vi "PhysioMoment.vi"() -> ()   [LabVIEW 2012]
doc: "Demonstrates general use of Obtain Queue, queues and the effects different settings have on queue behavior. It uses a queue to pass data between an Enqueue loop (producing data) and a Dequeue loop (consuming data). If both loops run at the same speed, the queue does not fill up.\n\nWhen the Enqueue loop runs fast and the Dequeue loop runs slow, the queue quickly fills up and the Enqueue loop must wait for the Dequeue loop to remove elements. If the Enqueue loop runs slow and the Dequeue loop runs fast, the queue is quickly emptied and the Dequeue loop must wait for the Enqueue loop to insert elements."
uses:
  global_variable/tvi_arx_ni9234_global.vi
  <vilib>/Utility/file.llb/Read From Spreadsheet File (I64).vi
  <vilib>/Utility/file.llb/Read From Spreadsheet File (DBL).vi
  <vilib>/Analysis/2dsp.llb/Decimate (continuous, DBL).vi
  <vilib>/Analysis/baseanly.llb/Mean (DBL).vi
  <vilib>/Utility/file.llb/Write To Spreadsheet File (DBL).vi
  <vilib>/Analysis/NI_AALBase.lvlib
  <vilib>/Analysis/NI_AALPro.lvlib
panel:
  in  "ECG":T1={"AMP."=1.0, "high cutoff"=0.0, "low cutoff"=0.0} {"low cutoff" format="%0.4f"; "high cutoff" format="%0.2f"}
  in  "LoadCell (4)":T1={"AMP."=1.0, "high cutoff"=0.0, "low cutoff"=0.0} {"low cutoff" format="%0.4f"; "high cutoff" format="%0.2f"}
  in  "LoadCell (3)":T1={"AMP."=1.0, "high cutoff"=0.0, "low cutoff"=0.0} {"low cutoff" format="%0.4f"; "high cutoff" format="%0.2f"}
  in  "LoadCell (2)":T1={"AMP."=1.0, "high cutoff"=0.0, "low cutoff"=0.0} {"low cutoff" format="%0.4f"; "high cutoff" format="%0.2f"}
  in  "LoadCell (1)":T1={"AMP."=1.0, "high cutoff"=0.0, "low cutoff"=0.0} {"low cutoff" format="%0.4f"; "high cutoff" format="%0.2f"}
  out "file length":i32=921600
  out "output data size":i32
  out "transfer data size":i32
  out "transfer data":csg[](array[numeric])
  in  "Tab Control 2":enum32{"Settings", "Main Panel"}(tab)
  in  "Hours":i32
  in  "minutes":i32=14
  in  "seconds":i32
  in  "Led Runner File":path=path "C:/Documents and Settings/nn4080/桌面/biofeedback system/control_file/led_pixel_7phase.txt"
  in  "Led Text File":path=path "C:/Documents and Settings/nn4080/桌面/biofeedback system/control_file/Led_like.txt"
  in  "Transfer Function":path=path "C:/Documents and Settings/nn4080/桌面/biofeedback system/control_file/FFT_512hzx10sec_modeling.txt"
  in  "Name":string
  out "ECG File":path=path "D:/PVDF-ACC-0102-1013.txt"
  out "GRF File":path=path "D:/PVDF-ACC-0102-1013.txt"
  out "CURRENT STEP INTERVAL (sec)":dbl format="%#_3g"
  out "Recording":bool
  out "Boolean 2":bool
  out "Hours":i32
  out "minutes":i32=30
  out "seconds":i32
  in  "stop":bool
  in  "Tab Control":enum32{"GRF", "Raw Data"}(tab)
  out "10 SLOPE INCREMENT":dbl format="%#_3g"
  out "10 STRIDE INCREMENT":dbl format="%#_3g"
  out "5 SLOPE INCREMENT":dbl format="%#_3g"
  out "5 STRIDE INCREMENT":dbl format="%#_3g"
  out "1 SLOPE INCREMENT":dbl format="%#_3g"
  out "1 STRIDE INCREMENT":dbl format="%#_3g"
  out "TVItv SCORE":dbl format="%#_3g"
  out "Slope SCORE":dbl format="%#_3g"
  out "TVItv SCORE":dbl format="%#_3g"
  out "Slope SCORE":dbl format="%#_3g"
  out "Slope SCORE":dbl format="%#_3g"
  out "TVItv SCORE":dbl format="%#_3g"
  out "Bio-Feedback System":bool[][](array[boolean])
  out "Right Foot GRF":cluster{dbl[], "Z-Score":dbl[]}[](graph)
  out "Left Foot GRF":cluster{dbl[], "Z-Score":dbl[]}[](graph)
  out "1 Stride":cluster{i32[], "Best Linear Fit":dbl[]}[](graph)
  out "5 Strides":cluster{i32[], "Best Linear Fit":dbl[]}[](graph)
  out "10 Strides":cluster{i32[], "Best Linear Fit":dbl[]}[](graph)
  out "GRF Output":dbl[](graph)
  out "GRF Input":cluster{dbl[], "Z-Score":dbl[]}[](graph)
  out "ECG":dbl[](graph)
  out "led loop execute time":dbl
  out "tvit (10 strides)":dbl
  out "tvit (10 strides)":dbl[](array[numeric])
  out "running phase":i8
  out "step-interval":dbl
  out "baseline value":dbl
  out "tvit array size\n(step count)":i32
  out "tvit (step)":dbl[](array[numeric])
  out "tvit (stride)":dbl
  out "tvit stride":dbl[](array[numeric])
  out "tvit stride array size":i32
  out "tvit (5 strides)":dbl[](array[numeric])
  out "tvit (5 strides)":dbl
  out "mean":dbl
  out "new step interval":dbl
  out "new step global index":dbl
  out "Tvit of new step":dbl
  out "step-index":dbl[](array[numeric])
  out "step-length":dbl[](array[numeric])
  out "vaild Tvit":dbl[](array[numeric])
  out "points per loop":i32
  out "GRF Input size":i32
  out "GRF Output size":i32
  out "main loop":i32
  out "std(loadcell)":dbl
  out "new step index(global) in last loop":dbl
  out "window start index":i32
  out "new step interval in last loop":dbl
  out "counter (sec)":string
  out "loop execution time":dbl
  out "zero-crossing point\n(increasing)":dbl[](array[numeric])
  out "area between zero-crossing points \n(z-score series)":dbl[](array[numeric])
  out "interval between \nzero-crossing points":dbl[](array[numeric])
  out "zero-crossing interval\nlower threshold":dbl
  out "step-index\n(in window)":dbl[](array[numeric])
  # "Ground Reaction Force \nBio-FeedBack System"
  # "Setting Time"
  # "Elapsed Time"
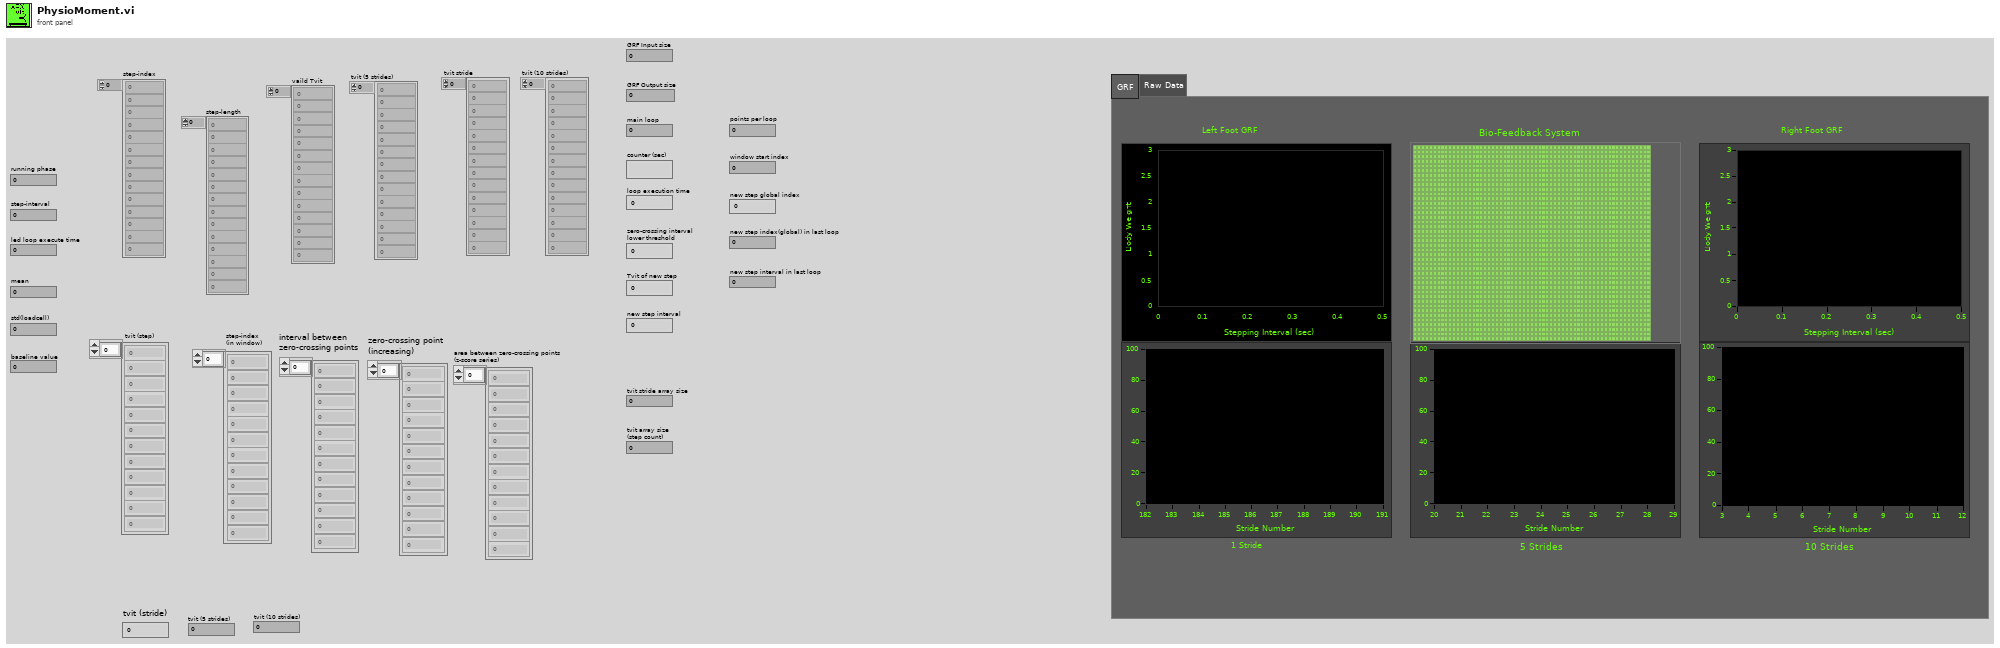
[diagram p1: front panel]
types:
  T1 = cluster{"AMP.":dbl, "high cutoff":dbl, "low cutoff":dbl}
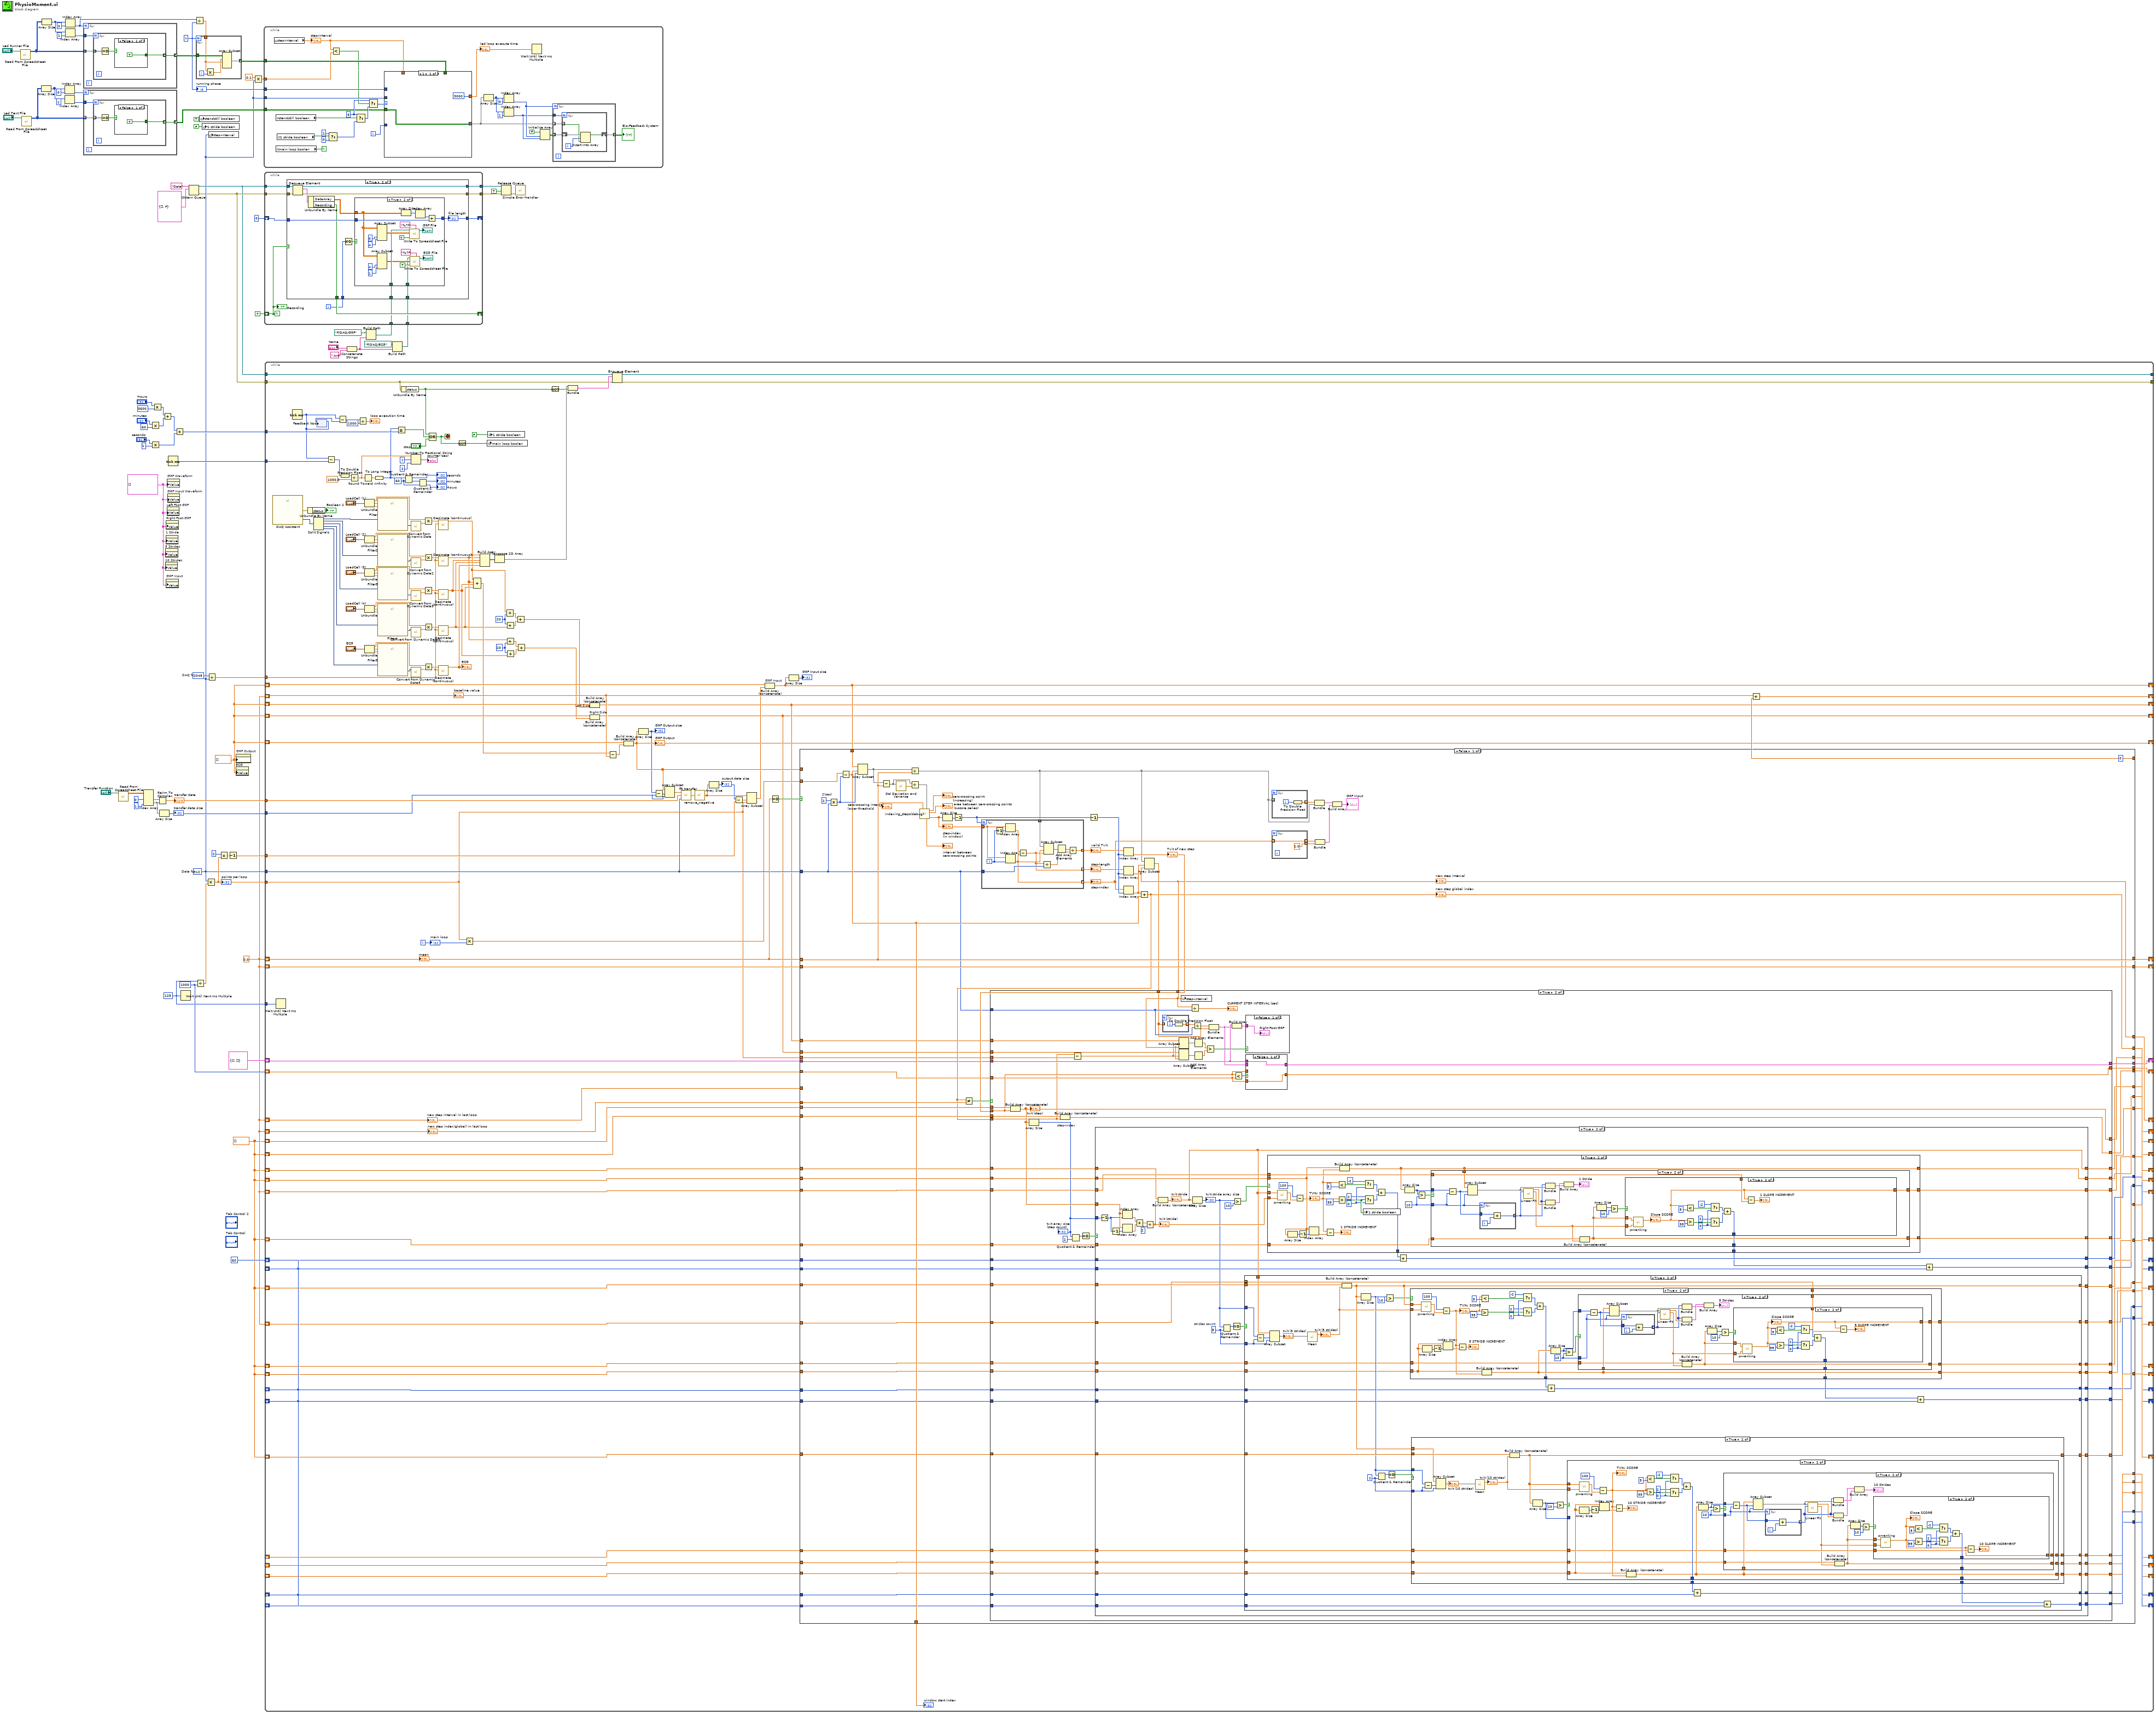
[diagram p0: block diagram]
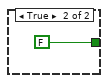
[diagram p4: hidden frame]
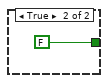
[diagram p5: hidden frame]
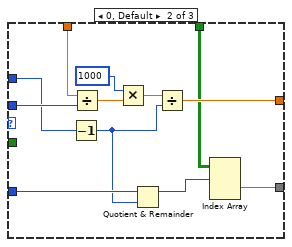
[diagram p6: hidden frame]
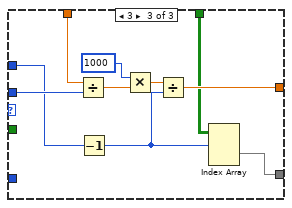
[diagram p7: hidden frame]
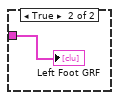
[diagram p10: hidden frame]
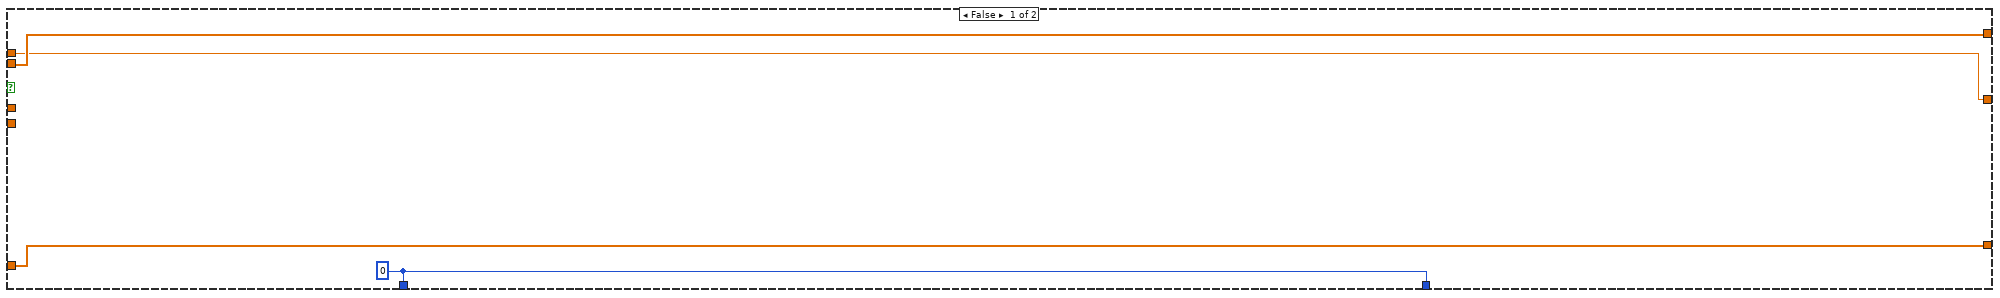
[diagram p12: hidden frame]
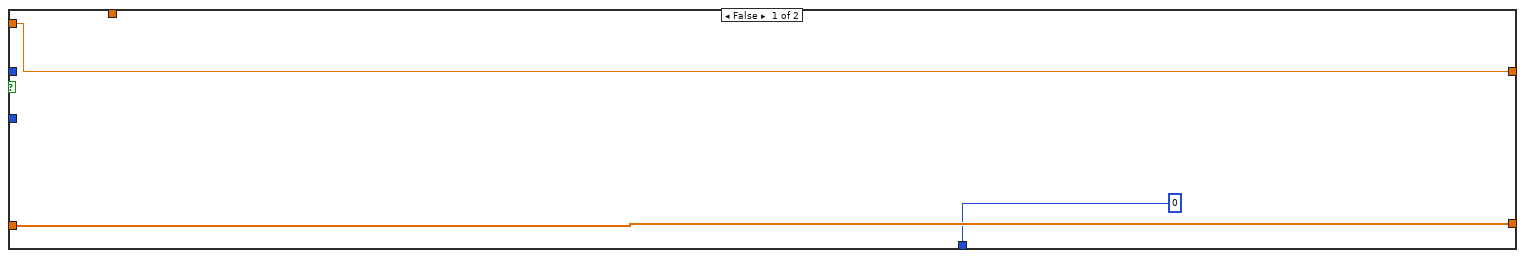
[diagram p13: hidden frame]
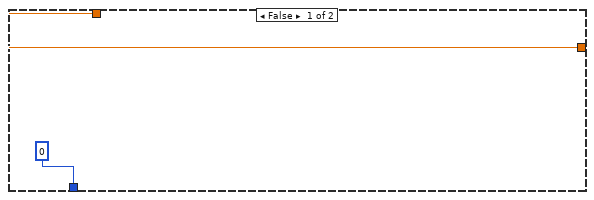
[diagram p14: hidden frame]
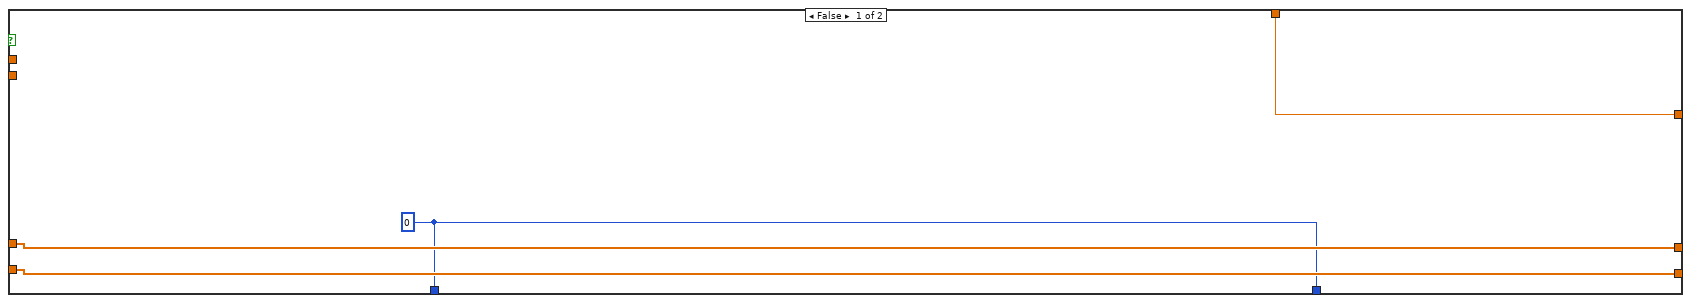
[diagram p16: hidden frame]
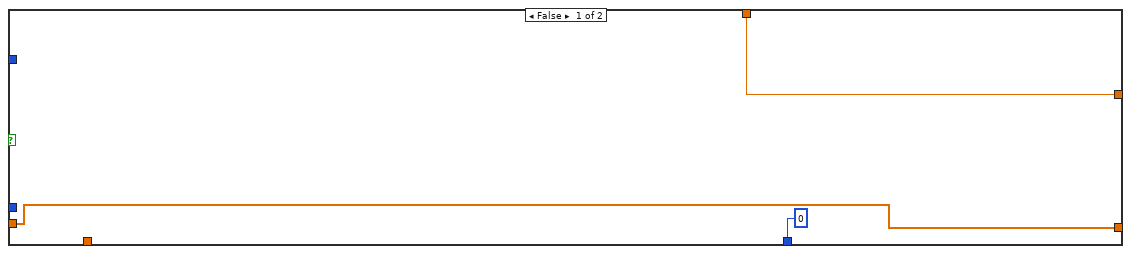
[diagram p17: hidden frame]
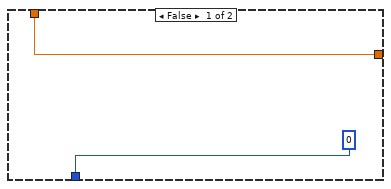
[diagram p18: hidden frame]
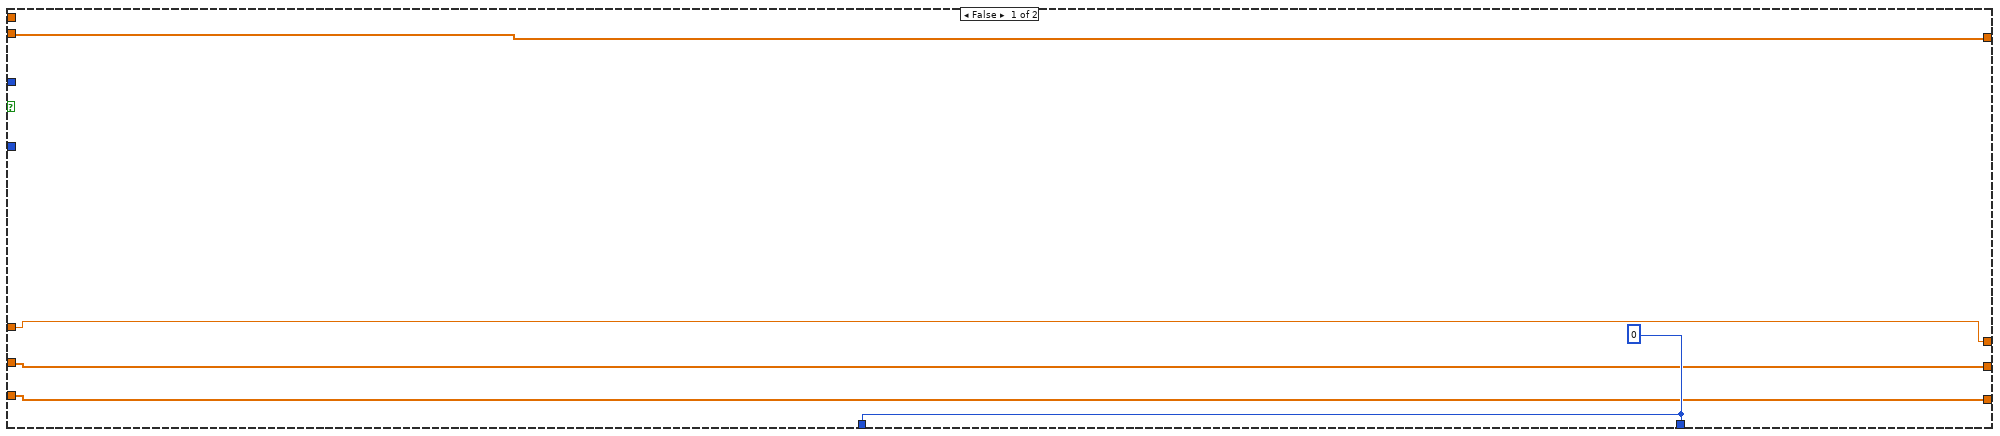
[diagram p19: hidden frame]
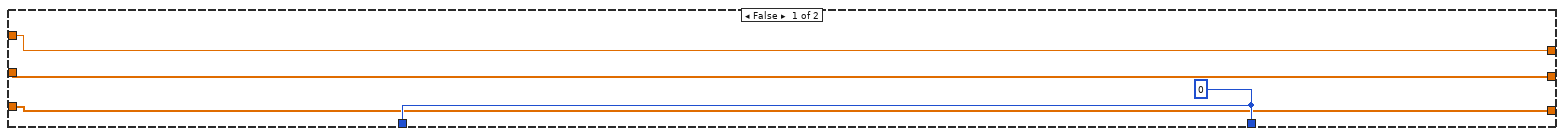
[diagram p20: hidden frame]
diagram:
  w9 = 2048  # DAQ fs
  w39 = 60
  (unwired) 1
  w41 = 7
  w1 = dbl[] []
  w4 = cluster{dbl[], "Z-Score":dbl[]}[] [] ("Z-Score Waveform (2 sec)")
  w2 = 0.0
  w8 = 512  # Data fs
  w3 = dbl[] []
  w31 = 1000
  w63 = u32 125 ("millisecond multiple")
  n1 = call-poly <vilib>:"Read From Spreadsheet File.vi"("file path (dialog if empty)"="Led Runner File") -> ("all rows"=w52:i64[][])  [unwired: 6 in, 4 out]
  n2 = call-poly <vilib>:"Read From Spreadsheet File.vi"("file path (dialog if empty)"="Led Text File") -> ("all rows"=w46:i64[][])  [unwired: 6 in, 4 out]
  n3 = Array Size(array=w46) -> (size(s)=w47:i32[])
  n4 = Array Size(array=w52) -> (size(s)=w51:i32[])
  n5 = Index Array(array=w47, index=0) -> (element=w45:i32)
  n6 = Index Array(array=w47) -> (element=w44:i32)  [unwired: 1 in]
  n7 = Index Array(array=w51, index=0) -> (element=w42:i32)
  n8 = Index Array(array=w51, index=1) -> (element=w55:i32)
  n9 = for {
    N: w42 -> [_]
    tunnel: w52 -> [w78] mode=indexing
    tunnel: [w77] -> w54 mode=indexing
    tunnel: w55 -> [w76]
    n10 = for {
      N: w76 -> [_]
      tunnel: w78 -> [w80] mode=indexing
      tunnel: [w79] -> w77 mode=indexing
      n11 = Equal To 0?(x=w80) -> (x = 0?=w81:bool)
      n12 = case shown="False" w81 {
        tunnel: [TRUE FALSE] -> w79
        frame False {
        }
        frame True {
        }
      }
    }
  }
  n13 = for {
    N: w45 -> [_]
    tunnel: w46 -> [w86] mode=indexing
    tunnel: [w85] -> w43 mode=indexing
    tunnel: w44 -> [w84]
    n14 = for {
      N: w84 -> [_]
      tunnel: w86 -> [w88] mode=indexing
      tunnel: [w87] -> w85 mode=indexing
      n15 = Equal To 0?(x=w88) -> (x = 0?=w89:bool)
      n16 = case shown="False" w89 {
        tunnel: [TRUE FALSE] -> w87
        frame False {
        }
        frame True {
        }
      }
    }
  }
  n17 = call-poly <vilib>:"Read From Spreadsheet File.vi"("file path (dialog if empty)"="Transfer Function") -> ("all rows"=w37:dbl[][])  [unwired: 6 in, 4 out]
  n18 = Index Array(array=w37, index (col) #1=0, index (col) #2=1) -> (element #1=w34:dbl[], element #2=w32:dbl[])  [unwired: 2 in]
  n19 = Multiply(x="minutes", y=60) -> (x*y=w75:i32)
  n20 = Multiply(x="seconds", y=1) -> (x*y=w66:i32)
  n21 = Multiply(x="Hours", y=3600) -> (x*y=w74:i32)
  n22 = Re/Im To Complex(1:w32, 2:w34) -> (0:w33:cdb[])
  "transfer data" <- w33
  n23 = Array Size(array=w32) -> (size(s)=w27:i32)
  "transfer data size" <- w27
  n24 = Add(x=w74, y=w75) -> (x+y=w67:i32)
  n25 = property on="10 Strides" class="XYGraph (strict)"("Value"=w4) -> ()  [unwired: 2 in, 2 out]
  n26 = property on="5 Strides" class="XYGraph (strict)"("Value"=w4) -> ()  [unwired: 2 in, 2 out]
  n27 = property on="1 Stride" class="XYGraph (strict)"("Value"=w4) -> ()  [unwired: 2 in, 2 out]
  n28 = property on="Right Foot GRF" class="XYGraph (strict)"("Value"=w4) -> ()  [unwired: 2 in, 2 out]
  n29 = property on="GRF Input" class="XYGraph (strict)"("Value"=w4) -> ()  [unwired: 2 in, 2 out]
  n30 = property on="Left Foot GRF" class="XYGraph (strict)"("Value"=w4) -> ()  [unwired: 2 in, 2 out]
  n31 = property on="GRF Waveform" class="XYGraph (strict)"("Value"=w4) -> ()  [unwired: 2 in, 2 out]
  n32 = property on="GRF Input Waveform" class="XYGraph (strict)"("Value"=w4) -> ()  [unwired: 2 in, 2 out]
  n33 = Tick Count (ms)() -> (millisecond timer value=w65:u32)
  n34 = Add(x=w67, y=w66) -> (x+y=w64:i32)
  n35 = Wait Until Next ms Multiple(millisecond multiple=w63) -> ()  [unwired: 1 out]
  n36 = Obtain Queue(name (unnamed)="Data", element data type=cluster{"DataArray":dbl[][], "Recording":bool} {"DataArray"=[], "Recording"=FALSE}) -> (queue out=w5:refnum<queue>, error out=w6:errorcluster)  [unwired: 3 in, 1 out]
  n37 = Divide(x=w42, y=w41) -> (x/y=w40:dbl)
  n38 = Divide(x=w63, y=w31) -> (x/y=w62:dbl)
  n39 = for {
    N: w41 -> [_]
    tunnel: w54 -> [w96]
    tunnel: w40 -> [w93]
    tunnel: [w94] -> w53 mode=indexing
    i -> [w95]
    n40 = Multiply(x=w93, y=w95) -> (x*y=w92:dbl)
    n41 = Array Subset(array=w96, index (row)=w92, length (row)=w93) -> (w94:bool[][])  [unwired: 2 in]
  }
  n42 = global write "tvi_arx_ni9234_global.vi" "standstill boolean"(TRUE) -> ()
  n43 = global write "tvi_arx_ni9234_global.vi" "1 stride boolean"(FALSE) -> ()
  n44 = Multiply(x=w8, y=w62) -> (x*y=w28:dbl)
  "points per loop" <- w28
  n45 = Divide(x=w9, y=w8) -> (x/y=w7:dbl)
  n46 = global write "tvi_arx_ni9234_global.vi" "step-interval"(w8) -> ()
  n47 = Multiply(x=2, y=w28) -> (x*y=w26:dbl)
  n48 = Decrement(x=w26) -> (x-1=w25:dbl)
  n49 = property on="GRF Output" class="WFChart (strict)"("History Data"=w3) -> ()  [unwired: 2 in, 2 out]
  n50 = property on="ECG" class="WFChart (strict)"("Value"=w3) -> ()  [unwired: 2 in, 2 out]
  n51 = Multiply(x=0.1, y=w8) -> (x*y=w49:dbl)
  n52 = while {
    tunnel: w53 -> [w118]
    tunnel: w8 -> [w116]
    tunnel: w41 -> [w119]
    tunnel: w49 -> [w103]
    tunnel: w43 -> [w98]
    i -> [w120]
    stop <- w123 continue-if-true
    w100 = 3
    n53 = global read "tvi_arx_ni9234_global.vi" "step-interval"() -> (w104:dbl)
    "step-interval" <- w104
    n54 = global read "tvi_arx_ni9234_global.vi" "standstill boolean"() -> (w114:bool)
    n55 = global read "tvi_arx_ni9234_global.vi" "main loop boolen"() -> (w123:bool)
    n56 = global read "tvi_arx_ni9234_global.vi" "1 stride boolean"() -> (w117:bool)
    n57 = Select(t=1, s=w117, f=0) -> (s? t:f=w97:i32)
    n58 = Less?(x=w104, y=w103) -> (x < y?=w102:bool)
    n59 = Select(t=w100, s=w114, f=w97) -> (s? t:f=w99:i32)
    n60 = Select(t=w100, s=w102, f=w99) -> (s? t:f=w101:i32)
    n61 = case shown="1" w101 {
      tunnel: w120 -> [_ w145 _]
      tunnel: w119 -> [_ w138 w149]
      tunnel: w118 -> [_ w136 w147]
      tunnel: w116 -> [_ w141 w151]
      tunnel: w104 -> [_ w140 w152]
      tunnel: [3000 w139 w150] -> w115
      tunnel: [w132 w134 w148] -> w105
      tunnel: w98 -> [w132 _ _]
      frame 1 {
      }
      frame 0, Default {
        n62 = Decrement(x=w138) -> (x-1=w137:i32)
        n63 = Divide(x=w140, y=w141) -> (x/y=w143:dbl)
        n64 = Multiply(x=1000, y=w143) -> (x*y=w144:dbl)
        n65 = Quotient & Remainder(x=w145, y=w137) -> (x-y*floor(x/y)=w135:i32)  [unwired: 1 out]
        n66 = Divide(x=w144, y=w137) -> (x/y=w139:dbl)
        n67 = Index Array(array=w136, index (dim 0)=w135) -> (element=w134:bool[][])  [unwired: 2 in]
      }
      frame 3 {
        n68 = Divide(x=w152, y=w151) -> (x/y=w154:dbl)
        n69 = Decrement(x=w149) -> (x-1=w146:i32)
        n70 = Multiply(x=1000, y=w154) -> (x*y=w155:dbl)
        n71 = Divide(x=w155, y=w146) -> (x/y=w150:dbl)
        n72 = Index Array(array=w147, index (dim 0)=w146) -> (element=w148:bool[][])  [unwired: 2 in]
      }
    }
    "led loop execute time" <- w115
    n73 = Array Size(array=w105) -> (size(s)=w108:i32[])
    n74 = Index Array(array=w108, index=0) -> (element=w107:i32)
    n75 = Index Array(array=w108, index=1) -> (element=w106:i32)
    n76 = Wait Until Next ms Multiple(millisecond multiple=w115) -> ()  [unwired: 1 out]
    n77 = Initialize Array(FALSE, w107, w106) -> (w112:bool[][])
    n78 = for {
      N: w107 -> [_]
      tunnel: [w127] -> w109 mode=indexing
      tunnel: w105 -> [w126] mode=indexing
      tunnel: w112 -> [w125] mode=indexing
      tunnel: w106 -> [w124]
      n79 = for {
        N: w124 -> [_]
        tunnel: w126 -> [w128] mode=indexing
        shift-right: [w131] -> w127
        shift-left: w125 -> [w129]
        i -> [w130]
        n80 = Insert Into Array(array=w129, index=w130, new element=w128) -> (w131:bool[])
      }
    }
    "Bio-Feedback System" <- w109
  }
  n81 = while {
    tunnel: w65 -> [w324]
    tunnel: w64 -> [w323]
    tunnel: w63 -> [w320]
    shift-right: [w282] -> _
    shift-left: w2 -> [w292]
    shift-right: [w281] -> _
    shift-left: w2 -> [w291]
    tunnel: w28 -> [w156]
    shift-right: [w243] -> _
    shift-left: w3 -> [w307]
    tunnel: w8 -> [w242]
    shift-right: [w286] -> _
    shift-left: w3 -> [w306]
    shift-right: [w302] -> _
    shift-left: w2 -> [w303]
    shift-right: [w301] -> _
    shift-left: w2 -> [w300]
    shift-right: [w285] -> _
    shift-left: w1 -> [w298]
    shift-right: [w284] -> _
    shift-left: w1 -> [w297]
    shift-right: [w296] -> _
    shift-left: w1 -> [w295]
    shift-right: [w294] -> _
    shift-left: w1 -> [w293]
    shift-right: [w288] -> _
    shift-left: w2 -> [w287]
    shift-right: [w279] -> _
    shift-left: w1 -> [w278]
    shift-right: [w276] -> _
    shift-left: w1 -> [w275]
    shift-right: [w274] -> _
    shift-left: w39 -> [w273]
    shift-right: [w272] -> _
    shift-left: w39 -> [w269]
    shift-right: [w271] -> _
    shift-left: w1 -> [w270]
    shift-right: [w268] -> _
    shift-left: w1 -> [w267]
    shift-right: [w266] -> _
    shift-left: w39 -> [w265]
    shift-right: [w262] -> _
    shift-left: w39 -> [w261]
    shift-right: [w264] -> _
    shift-left: w1 -> [w263]
    shift-right: [w260] -> _
    shift-left: w39 -> [w254]
    shift-right: [w259] -> _
    shift-left: _ -> [w258]
    shift-right: [w257] -> _
    shift-left: _ -> [w256]
    shift-right: [w255] -> _
    shift-left: w39 -> [w253]
    shift-right: [w252] -> _
    shift-left: _ -> [w251]
    shift-right: [w250] -> _
    shift-left: w2 -> [w249]
    shift-right: [w248] -> _
    shift-left: w2 -> [w247]
    tunnel: w33 -> [w244]
    tunnel: w27 -> [w238]
    shift-right: [w223] -> _
    shift-left: w3 -> [w227]
    shift-right: [w222] -> _
    shift-left: w3 -> [w226]
    shift-right: [w218] -> _
    shift-left: cluster{dbl[], dbl[]} {[], []} -> [w221]
    shift-right: [w219] -> _
    shift-left: w31 -> [w220]
    tunnel: w25 -> [w217]
    tunnel: w7 -> [w170]
    tunnel: [w163] -> _
    tunnel: [w162] -> _
    tunnel: w5 -> [w159]
    tunnel: w6 -> [w158]
    i -> [w157]
    stop <- w283 stop-if-true
    w228 = 20
    w229 = 20
    w299 = 60 ("floor(x/y)")
    n82 = call "DAQ Assistant"() -> ("data"=w201:dynamicdata, "error out"=w216:errorcluster)  [unwired: 16 in, 2 out]
    n83 = Wait Until Next ms Multiple(millisecond multiple=w320) -> ()  [unwired: 1 out]
    n84 = Tick Count (ms)() -> (millisecond timer value=w311:u32)
    n85 = Unbundle By Name(w216) -> ("status"=→"Boolean 2":bool)
    n86 = Split Signals(w201) -> (w200:dynamicdata, w199:dynamicdata, w176:dynamicdata, w175:dynamicdata, w174:dynamicdata)  [unwired: 5 in]
    n87 = feedback-in #1(w311) -> ()
    n88 = feedback #1() -> (w316:u32)  [unwired: 1 in]
    n89 = Subtract(x=w311, y=w324) -> (x-y=w326:u32)
    n90 = Subtract(x=w311, y=w316) -> (x-y=w319:u32)
    n91 = To Double Precision Float(number=w326) -> (double precision float=w327:dbl)
    n92 = Divide(x=w327, y=1000.0) -> (x/y=w312:dbl)
    n93 = Divide(x=w319, y=1000) -> (x/y=→"loop execution time":dbl)
    n94 = Round Toward -Infinity(1:w312) -> (0:w325:dbl)
    n95 = Unbundle("LoadCell (1)") -> ("AMP."=w207:dbl, "high cutoff"=w213:dbl, "low cutoff"=w212:dbl)
    n96 = Unbundle("LoadCell (2)") -> ("AMP."=w204:dbl, "high cutoff"=w211:dbl, "low cutoff"=w210:dbl)
    n97 = Unbundle("LoadCell (3)") -> ("AMP."=w188:dbl, "high cutoff"=w194:dbl, "low cutoff"=w193:dbl)
    n98 = Unbundle("LoadCell (4)") -> ("AMP."=w185:dbl, "high cutoff"=w192:dbl, "low cutoff"=w191:dbl)
    n99 = Unbundle("ECG") -> ("AMP."=w173:dbl, "high cutoff"=w181:dbl, "low cutoff"=w180:dbl)
    n100 = To Long Integer(number=w325) -> (32bit integer=w309:i32)
    n101 = call "Filter"("Lower Cut-Off"=w212, "Upper Cut-Off"=w213, "Signal"=w200) -> ("Filtered Signal"=w209:dynamicdata)  [unwired: 7 in, 1 out]
    n102 = call "Filter2"("Lower Cut-Off"=w210, "Upper Cut-Off"=w211, "Signal"=w199) -> ("Filtered Signal"=w205:dynamicdata)  [unwired: 7 in, 1 out]
    n103 = call "Filter3"("Lower Cut-Off"=w193, "Upper Cut-Off"=w194, "Signal"=w176) -> ("Filtered Signal"=w190:dynamicdata)  [unwired: 7 in, 1 out]
    n104 = call "Filter4"("Lower Cut-Off"=w191, "Upper Cut-Off"=w192, "Signal"=w175) -> ("Filtered Signal"=w186:dynamicdata)  [unwired: 7 in, 1 out]
    n105 = call "Filter5"("Lower Cut-Off"=w180, "Upper Cut-Off"=w181, "Signal"=w174) -> ("Filtered Signal"=w178:dynamicdata)  [unwired: 7 in, 1 out]
    n106 = Greater Or Equal?(x=w309, y=w323) -> (x >= y?=w322:bool)
    n107 = Unbundle By Name(w158) -> ("status"=w160:bool)
    n108 = Quotient & Remainder(x=w309, y=w299) -> (x-y*floor(x/y)=→"seconds":i32, floor(x/y)=w328:i32)
    n109 = call "Convert from Dynamic Data"("Dynamic Data Type"=w209) -> ("Array"=w208:dbl[])  [unwired: 3 in]
    n110 = call "Convert from Dynamic Data2"("Dynamic Data Type"=w205) -> ("Array"=w206:dbl[])  [unwired: 3 in]
    n111 = call "Convert from Dynamic Data3"("Dynamic Data Type"=w190) -> ("Array"=w189:dbl[])  [unwired: 3 in]
    n112 = call "Convert from Dynamic Data4"("Dynamic Data Type"=w186) -> ("Array"=w187:dbl[])  [unwired: 3 in]
    n113 = call "Convert from Dynamic Data5"("Dynamic Data Type"=w178) -> ("Array"=w179:dbl[])  [unwired: 3 in]
    n114 = Number To Fractional String(number=w312, width (-)=7, precision (6)=2) -> (F-format string=→"counter (sec)":string)  [unwired: 1 in]
    n115 = Quotient & Remainder(x=w328, y=w299) -> (x-y*floor(x/y)=→"minutes":i32, floor(x/y)=→"Hours":i32)
    n116 = Multiply(x=w207, y=w208) -> (x*y=w198:dbl[])
    n117 = Multiply(x=w188, y=w189) -> (x*y=w184:dbl[])
    n118 = Multiply(x=w204, y=w206) -> (x*y=w197:dbl[])
    n119 = Multiply(x=w185, y=w187) -> (x*y=w183:dbl[])
    n120 = Multiply(x=w173, y=w179) -> (x*y=w177:dbl[])
    n121 = Compound Arithmetic op=OR(w160, w322, "stop") -> (w283:bool)
    n122 = call-poly <vilib>:"Decimate (continuous).vi"("decimating factor"=w170, "X"=w198) -> ("Decimated Array"=w168:dbl[])  [unwired: 8 in, 1 out]
    n123 = call-poly <vilib>:"Decimate (continuous).vi"("decimating factor"=w170, "X"=w197) -> ("Decimated Array"=w167:dbl[])  [unwired: 8 in, 1 out]
    n124 = call-poly <vilib>:"Decimate (continuous).vi"("decimating factor"=w170, "X"=w184) -> ("Decimated Array"=w166:dbl[])  [unwired: 8 in, 1 out]
    n125 = call-poly <vilib>:"Decimate (continuous).vi"("decimating factor"=w170, "X"=w183) -> ("Decimated Array"=w169:dbl[])  [unwired: 8 in, 1 out]
    n126 = call-poly <vilib>:"Decimate (continuous).vi"("decimating factor"=w170, "X"=w177) -> ("Decimated Array"=w172:dbl[])  [unwired: 8 in, 1 out]
    "ECG" <- w172
    n127 = Not(x=w283) -> (.not. x?=w280:bool)
    n128 = Multiply(x=w156, y=w157) -> (x*y=w241:dbl)
    n129 = Compound Arithmetic op=ADD(w168, w167, w166, w169) -> (w171:dbl[])
    n130 = Build Array(w168, w167, w166, w169, w172) -> (w202:dbl[][])
    n131 = global write "tvi_arx_ni9234_global.vi" "main loop boolen"(w280) -> ()
    n132 = global write "tvi_arx_ni9234_global.vi" "1 stride boolean"(FALSE) -> ()
    n133 = Transpose 2D Array(2D array=w202) -> (transposed array=w161:dbl[][])
    n134 = Add(x=w168, y=w228) -> (x+y=w231:dbl[])
    n135 = Add(x=w228, y=w169) -> (x+y=w230:dbl[])
    n136 = Add(x=w167, y=w229) -> (x+y=w233:dbl[])
    n137 = Add(x=w229, y=w166) -> (x+y=w232:dbl[])
    n138 = Add(x=w231, y=w230) -> (x+y=w225:dbl[])
    n139 = Add(x=w233, y=w232) -> (x+y=w224:dbl[])
    n140 = Not(x=w160) -> (.not. x?=w165:bool)
    n141 = Bundle(w161, w165) -> (w164:cluster{dbl[][], bool})  [unwired: 1 in]
    n142 = Build Array (concatenate) "Right Side"(w226, w224) -> (w222:dbl[])
    n143 = Build Array (concatenate) "Left Side"(w227, w225) -> (w223:dbl[])
    n144 = Subtract(x=w171, y=w287) -> (x-y=w290:dbl[])
    n145 = Enqueue Element(queue=w159, element=w164, error in (no error)=w158) -> (queue out=w163:refnum<queue>, error out=w162:errorcluster)  [unwired: 1 in, 1 out]
    n146 = Build Array (concatenate)(w307, w290) -> (w243:dbl[])
    "GRF Output" <- w243
    n147 = Array Size(array=w243) -> (size(s)=w239:i32)
    "GRF Output size" <- w239
    n148 = Subtract(x=w239, y=w238) -> (x-y=w240:i32)
    n149 = Array Subset(array=w243, index=w240, length=w238) -> (w246:dbl[])
    n150 = call "fft_transfer.vi"("Sample Rate"=w242, "Transfer Function"=w244, "GRF Output"=w246) -> ("GRF Input"=w245:dbl[])
    n151 = call "remove_negative.vi"("input array"=w245) -> ("output array"=w237:dbl[])
    n152 = Array Size(array=w237) -> (size(s)=w236:i32)
    "output data size" <- w236
    n153 = Subtract(x=w236, y=w217) -> (x-y=w235:dbl)
    n154 = Array Subset(array=w237, index=w235, length=w156) -> (w234:dbl[])
    n155 = Build Array (concatenate) "GRF Input"(w306, w234) -> (w286:dbl[])
    n156 = Equal To 0?(x=w300) -> (x = 0?=w308:bool)
    n157 = Array Size(array=w286) -> (size(s)=→"GRF Input size":i32)
    n158 = case shown="False" w308 {
      tunnel: w300 -> [w380 w943]
      tunnel: [w402 w926] -> w305
      tunnel: w242 -> [w370 w904]
      tunnel: w241 -> [w415 w924]
      tunnel: w243 -> [_ w932]
      tunnel: w303 -> [w391 w947]
      tunnel: [w391 w930] -> w302
      tunnel: [w371 w934] -> w282
      tunnel: [w375 w935] -> w281
      tunnel: [w380 w942] -> w301
      tunnel: w292 -> [w399 w934]
      tunnel: [w333 w939] -> w285
      tunnel: w298 -> [w398 w939]
      tunnel: [w397 w938] -> w284
      tunnel: w297 -> [w396 w938]
      tunnel: [w395 w937] -> w296
      tunnel: w295 -> [w394 w937]
      tunnel: [w393 w936] -> w294
      tunnel: w293 -> [w392 w936]
      tunnel: w291 -> [_ w935]
      tunnel: w286 -> [w389 w927]
      tunnel: [0 w925] -> w289
      tunnel: [w374 w923] -> w279
      tunnel: w278 -> [w373 w923]
      tunnel: [w369 w922] -> w276
      tunnel: w275 -> [w368 w922]
      tunnel: [w367 w920] -> w274
      tunnel: w273 -> [w366 w920]
      tunnel: [w365 w919] -> w272
      tunnel: [w364 w921] -> w271
      tunnel: w270 -> [w363 w921]
      tunnel: w269 -> [w362 w919]
      tunnel: [w361 w913] -> w268
      tunnel: w267 -> [w360 w913]
      tunnel: [w359 w912] -> w266
      tunnel: w265 -> [w358 w912]
      tunnel: [w357 w914] -> w264
      tunnel: w263 -> [w356 w914]
      tunnel: [w355 w911] -> w262
      tunnel: w261 -> [w354 w911]
      tunnel: [w353 w916] -> w260
      tunnel: [w352 w917] -> w259
      tunnel: w258 -> [w351 w917]
      tunnel: [w350 w918] -> w257
      tunnel: w256 -> [w349 w918]
      tunnel: [w348 w915] -> w255
      tunnel: w254 -> [w347 w916]
      tunnel: w253 -> [w346 w915]
      tunnel: [w345 w908] -> w252
      tunnel: w251 -> [w344 w908]
      tunnel: [w343 w909] -> w250
      tunnel: w249 -> [w342 w909]
      tunnel: [w341 w910] -> w248
      tunnel: w247 -> [w340 w910]
      tunnel: w223 -> [w339 _]
      tunnel: w222 -> [w338 _]
      tunnel: w221 -> [w337 w907]
      tunnel: w220 -> [w336 w906]
      tunnel: [w335 w906] -> w219
      tunnel: [w334 w907] -> w218
      tunnel: w156 -> [w332 _]
      frame False {
        w409 = 2  # 2(sec)
        n159 = Multiply(x=w409, y=w370) -> (x*y=w414:i32)
        n160 = Subtract(x=w415, y=w414) -> (x-y=w402:dbl)
        n161 = Array Subset(array=w389, index=w402, length=w414) -> (w377:dbl[])
        n162 = Subtract(x=w377, y=w380) -> (x-y=w378:dbl[])
        n163 = call <vilib>:"Std Deviation and Variance.vi"("X"=w378) -> ("standard deviation"=w416:dbl)  [unwired: 1 in, 2 out]
        n164 = Divide(x=w377, y=w380) -> (x/y=w376:dbl[])
        n165 = Divide(x=w378, y=w416) -> (x/y=w379:dbl[])
        n166 = call "indexing_steps(debug).vi"("z-score series (input)"=w379) -> ("lower threshold of zeros-interval"=→"zero-crossing interval\nlower threshold":dbl, "zeros-interval\n(interval between zero-crossing index)"=→"interval between \nzero-crossing points":dbl[], "increasing\nzero-crossing index"=→"zero-crossing point\n(increasing)":dbl[], "area between zero-crossing index"=→"area between zero-crossing points \n(z-score series)":dbl[], "index of steps (output)"=w407:dbl[])  [unwired: 1 in]
        "step-index\n(in window)" <- w407
        n167 = Array Size(array=w407) -> (size(s)=w408:i32)
        n168 = Decrement(x=w408) -> (x-1=w405:i32)
        n169 = for {
          N: w405 -> [_]
          tunnel: w407 -> [w896]
          tunnel: w376 -> [w899]
          tunnel: [w893] -> w404 mode=indexing
          tunnel: [w891] -> w403 mode=indexing
          tunnel: [w894] -> w382 mode=indexing
          tunnel: w370 -> [w895]
          i -> [w901]
          n170 = Increment(x=w901) -> (x+1=w902:i32)
          n171 = Index Array(array=w896, index=w902) -> (element=w900:dbl)
          n172 = Index Array(array=w896, index=w901) -> (element=w894:dbl)
          n173 = Subtract(x=w900, y=w894) -> (x-y=w891:dbl)
          n174 = Divide(x=w891, y=w895) -> (x/y=w892:dbl)
          n175 = Array Subset(array=w899, index=w894, length=w891) -> (w897:dbl[])
          n176 = Add Array Elements(numeric array=w897) -> (sum=w898:dbl)
          n177 = Divide(x=w898, y=w892) -> (x/y=w893:dbl)
        }
        "vaild Tvit" <- w404
        "step-length" <- w403
        "step-index" <- w382
        n178 = Decrement(x=w405) -> (x-1=w406:i32)
        n179 = Index Array(array=w404, index=w406) -> (element=w390:dbl)
        "Tvit of new step" <- w390
        n180 = Index Array(array=w403, index=w406) -> (element=w375:dbl)
        "new step interval" <- w375
        n181 = Index Array(array=w382, index=w406) -> (element=w401:dbl)
        n182 = Add(x=w401, y=w402) -> (x+y=w371:dbl)
        "new step global index" <- w371
        n183 = Not Equal?(x=w371, y=w399) -> (x != y?=w400:bool)
        n184 = Array Subset(array=w376, index=w401, length=w375) -> (w372:dbl[])
        n185 = case shown="True" w400 {
          tunnel: [w442 w498] -> w333
          tunnel: w398 -> [w442 w507]
          tunnel: w390 -> [_ w455]
          tunnel: [w440 w506] -> w397
          tunnel: w396 -> [w440 w505]
          tunnel: [w441 w504] -> w395
          tunnel: w394 -> [w441 w503]
          tunnel: [w439 w502] -> w393
          tunnel: w392 -> [w439 w501]
          tunnel: w375 -> [_ w452]
          tunnel: [w438 w500] -> w374
          tunnel: w373 -> [w438 w499]
          tunnel: w372 -> [_ w450]
          tunnel: w371 -> [_ w445]
          tunnel: w370 -> [_ w458]
          tunnel: [w437 w496] -> w369
          tunnel: w368 -> [w437 w495]
          tunnel: [w435 w494] -> w367
          tunnel: w366 -> [w435 w493]
          tunnel: [w434 w492] -> w365
          tunnel: [w436 w491] -> w364
          tunnel: w363 -> [w436 w490]
          tunnel: w362 -> [w434 w489]
          tunnel: [w432 w488] -> w361
          tunnel: w360 -> [w432 w487]
          tunnel: [w431 w486] -> w359
          tunnel: w358 -> [w431 w485]
          tunnel: [w433 w484] -> w357
          tunnel: w356 -> [w433 w483]
          tunnel: [w430 w482] -> w355
          tunnel: w354 -> [w430 w481]
          tunnel: [w427 w480] -> w353
          tunnel: [w428 w479] -> w352
          tunnel: w351 -> [w428 w478]
          tunnel: [w429 w477] -> w350
          tunnel: w349 -> [w429 w476]
          tunnel: [w426 w475] -> w348
          tunnel: w347 -> [w427 w474]
          tunnel: w346 -> [w426 w473]
          tunnel: [w423 w472] -> w345
          tunnel: w344 -> [w423 w471]
          tunnel: [w424 w470] -> w343
          tunnel: w342 -> [w424 w469]
          tunnel: [w425 w468] -> w341
          tunnel: w340 -> [w425 w467]
          tunnel: w339 -> [_ w461]
          tunnel: w338 -> [_ w460]
          tunnel: w337 -> [w422 w447]
          tunnel: w336 -> [w421 w454]
          tunnel: [w421 w456] -> w335
          tunnel: [w422 w449] -> w334
          tunnel: w332 -> [_ w443]
          frame False {
          }
          frame True {
            n186 = Build Array (concatenate)(w507, w455) -> (w498:dbl[])
            "tvit (step)" <- w498
            n187 = Array Size(array=w498) -> (size(s)=w497:i32)
            "tvit array size\n(step count)" <- w497
            n188 = Build Array (concatenate) "step-index"(w505, w445) -> (w506:dbl[])
            n189 = Quotient & Remainder(x=w497, y=2) -> (x-y*floor(x/y)=w510:i32)  [unwired: 1 out]
            n190 = Subtract(x=w445, y=w443) -> (x-y=w444:dbl)
            n191 = Equal To 0?(x=w510) -> (x = 0?=w508:bool)
            n192 = case shown="True" w508 {
              tunnel: w498 -> [_ w586]
              tunnel: [w535 w571] -> w504
              tunnel: w497 -> [_ w585]
              tunnel: [w536 w578] -> w502
              tunnel: w503 -> [w535 w577]
              tunnel: w501 -> [w536 w576]
              tunnel: [w534 w575] -> w500
              tunnel: w499 -> [w534 w574]
              tunnel: [w533 w567] -> w496
              tunnel: w495 -> [w533 w568]
              tunnel: [w531 w564] -> w494
              tunnel: w493 -> [w531 w565]
              tunnel: [w530 w563] -> w492
              tunnel: [w532 w558] -> w491
              tunnel: w490 -> [w532 w559]
              tunnel: w489 -> [w530 w562]
              tunnel: [w528 w561] -> w488
              tunnel: w487 -> [w528 w560]
              tunnel: [w527 w556] -> w486
              tunnel: w485 -> [w527 w555]
              tunnel: [w529 w554] -> w484
              tunnel: w483 -> [w529 w553]
              tunnel: [w526 w552] -> w482
              tunnel: w481 -> [w526 w551]
              tunnel: [w523 w550] -> w480
              tunnel: [w524 w549] -> w479
              tunnel: w478 -> [w524 w548]
              tunnel: [w525 w547] -> w477
              tunnel: w476 -> [w525 w546]
              tunnel: [w522 w545] -> w475
              tunnel: w474 -> [w523 w544]
              tunnel: w473 -> [w522 w543]
              tunnel: [w519 w542] -> w472
              tunnel: w471 -> [w519 w541]
              tunnel: [w520 w540] -> w470
              tunnel: w469 -> [w520 w539]
              tunnel: [w521 w538] -> w468
              tunnel: w467 -> [w521 w537]
              frame False {
              }
              frame True {
                w587 = 5  # strides count
                n193 = Decrement(x=w585) -> (x-1=w583:i32)
                n194 = Decrement(x=w583) -> (x-1=w584:i32)
                n195 = Index Array(array=w586, index=w583) -> (element=w581:dbl)
                n196 = Index Array(array=w586, index=w584) -> (element=w582:dbl)
                n197 = Add(x=w581, y=w582) -> (x+y=w580:dbl)
                n198 = Divide(x=w580, y=2) -> (x/y=w572:dbl)
                "tvit (stride)" <- w572
                n199 = Build Array (concatenate)(w577, w572) -> (w571:dbl[])
                "tvit stride" <- w571
                n200 = Array Size(array=w571) -> (size(s)=w569:i32)
                "tvit stride array size" <- w569
                n201 = Quotient & Remainder(x=w569, y=w587) -> (x-y*floor(x/y)=w588:i32)  [unwired: 1 out]
                n202 = Equal To 0?(x=w588) -> (x = 0?=w589:bool)
                n203 = Greater?(x=w569, y=10) -> (0:w573:bool)
                n204 = case shown="True" w589 {
                  tunnel: w587 -> [_ w713]
                  tunnel: w571 -> [_ w715]
                  tunnel: w569 -> [_ w712]
                  tunnel: [w676 w706] -> w578
                  tunnel: w576 -> [w676 w710]
                  tunnel: [w675 w705] -> w575
                  tunnel: w574 -> [w675 w704]
                  tunnel: [w673 w700] -> w561
                  tunnel: w560 -> [w673 w699]
                  tunnel: [w672 w694] -> w556
                  tunnel: w555 -> [w672 w697]
                  tunnel: [w674 w696] -> w554
                  tunnel: w553 -> [w674 w695]
                  tunnel: [w671 w693] -> w552
                  tunnel: w551 -> [w671 w691]
                  tunnel: [w668 w687] -> w550
                  tunnel: [w669 w689] -> w549
                  tunnel: w548 -> [w669 w688]
                  tunnel: [w670 w686] -> w547
                  tunnel: w546 -> [w670 w685]
                  tunnel: [w667 w683] -> w545
                  tunnel: w544 -> [w668 w682]
                  tunnel: w543 -> [w667 w681]
                  tunnel: [w666 w680] -> w542
                  tunnel: w541 -> [w666 w679]
                  tunnel: [w665 w678] -> w540
                  tunnel: w539 -> [w665 w677]
                  frame False {
                  }
                  frame True {
                    w707 = 2
                    n205 = Subtract(x=w712, y=w713) -> (x-y=w714:i32)
                    n206 = Array Subset(array=w715, index=w714, length=w713) -> (w716:dbl[])
                    "tvit (5 strides)" <- w716
                    n207 = call-poly <vilib>:"Mean.vi"("X"=w716) -> ("mean"=w711:dbl)  [unwired: 1 out]
                    "tvit (5 strides)" <- w711
                    n208 = Build Array (concatenate)(w710, w711) -> (w706:dbl[])
                    n209 = Array Size(array=w706) -> (size(s)=w701:i32)
                    n210 = Quotient & Remainder(x=w701, y=w707) -> (x-y*floor(x/y)=w709:i32)  [unwired: 1 out]
                    n211 = Greater?(x=w701, y=10) -> (0:w703:bool)
                    n212 = Equal To 0?(x=w709) -> (x = 0?=w708:bool)
                    n213 = case shown="True" w703 {
                      tunnel: w711 -> [_ w749]
                      tunnel: w706 -> [_ w745]
                      tunnel: [w719 w730] -> w700
                      tunnel: w699 -> [w719 w725]
                      tunnel: [w718 w729] -> w698
                      tunnel: [w720 w728] -> w696
                      tunnel: w695 -> [w720 w727]
                      tunnel: [w718 w726] -> w692
                      tunnel: [w717 w724] -> w678
                      tunnel: w677 -> [w717 w723]
                      frame False {
                        w718 = 0
                      }
                      frame True {
                        w731 = 10
                        w740 = 0
                        n214 = call "pr-ranking.vi"("element"=w749, "Database Array"=w745) -> ("PR Value"=w741:dbl)  [unwired: 1 out]
                        n215 = Array Size(array=w725) -> (size(s)=w744:i32)
                        n216 = Decrement(x=w744) -> (x-1=w743:i32)
                        n217 = Subtract(x=100, y=w741) -> (x-y=w722:dbl)
                        "TVItv SCORE" <- w722
                        n218 = Index Array(array=w725, index=w743) -> (element=w742:dbl)
                        n219 = Subtract(x=w722, y=w742) -> (x-y=→"5 STRIDE INCREMENT":dbl)
                        n220 = Greater?(x=w722, y=95) -> (0:w734:bool)
                        n221 = Less?(x=w722, y=5) -> (x < y?=w735:bool)
                        n222 = Build Array (concatenate)(w725, w722) -> (w730:dbl[])
                        n223 = Select(t=-2, s=w735, f=w740) -> (s? t:f=w737:i32)
                        n224 = Select(t=2, s=w734, f=w740) -> (s? t:f=w736:i32)
                        n225 = Add(x=w737, y=w736) -> (x+y=w729:i32)
                        n226 = Array Size(array=w730) -> (size(s)=w732:i32)
                        n227 = Greater?(x=w732, y=w731) -> (0:w733:bool)
                        n228 = case shown="True" w733 {
                          tunnel: w732 -> [_ w765]
                          tunnel: w731 -> [_ w764]
                          tunnel: w730 -> [_ w763]
                          tunnel: [w751 w758] -> w728
                          tunnel: w727 -> [w751 w756]
                          tunnel: [0 w757] -> w726
                          tunnel: [w750 w755] -> w724
                          tunnel: w723 -> [w750 w754]
                          frame False {
                          }
                          frame True {
                            n229 = Subtract(x=w765, y=w764) -> (x-y=w771:i32)
                            n230 = Array Subset(array=w763, index=w771, length=w764) -> (w770:dbl[])
                            n231 = for {
                              N: w764 -> [_]
                              tunnel: w771 -> [w790]
                              tunnel: [w789] -> w762 mode=indexing
                              i -> [w791]
                              n232 = Add(x=w790, y=w791) -> (x+y=w789:i32)
                            }
                            n233 = call <vilib>:"Linear Fit.vi"("Y"=w770, "X"=w762) -> ("Best Linear Fit"=w769:dbl[], "slope"=w753:dbl)  [unwired: 9 in, 3 out]
                            n234 = Bundle(w762, w770) -> (w767:cluster{i32[], dbl[]})  [unwired: 1 in]
                            n235 = Bundle(w762, "Best Linear Fit"=w769) -> (w768:cluster{i32[], "Best Linear Fit":dbl[]})  [unwired: 1 in]
                            n236 = Build Array (concatenate)(w756, w753) -> (w758:dbl[])
                            n237 = Build Array(w768, w767) -> (→"5 Strides":cluster{i32[], "Best Linear Fit":dbl[]}[])
                            n238 = Array Size(array=w758) -> (size(s)=w761:i32)
                            n239 = Greater?(x=w761, y=10) -> (0:w759:bool)
                            n240 = case shown="True" w759 {
                              tunnel: w758 -> [_ w788]
                              tunnel: w753 -> [_ w777]
                              tunnel: [0 w778] -> w757
                              tunnel: [w772 w775] -> w755
                              tunnel: w754 -> [w772 w776]
                              frame False {
                              }
                              frame True {
                                w785 = 0
                                n241 = call "pr-ranking.vi"("element"=w777, "Database Array"=w788) -> ("PR Value"=w775:dbl)  [unwired: 1 out]
                                "Slope SCORE" <- w775
                                n242 = Less?(x=w775, y=5) -> (x < y?=w780:bool)
                                n243 = Greater?(x=w775, y=95) -> (0:w779:bool)
                                n244 = Select(t=-2, s=w780, f=w785) -> (s? t:f=w782:i32)
                                n245 = Select(t=2, s=w779, f=w785) -> (s? t:f=w781:i32)
                                n246 = Add(x=w782, y=w781) -> (x+y=w778:i32)
                                n247 = Subtract(x=w775, y=w776) -> (x-y=→"5 SLOPE INCREMENT":dbl)
                              }
                            }
                          }
                        }
                      }
                    }
                    n248 = case shown="True" w708 {
                      tunnel: w707 -> [_ w812]
                      tunnel: w701 -> [_ w811]
                      tunnel: w706 -> [_ w810]
                      tunnel: [w796 w806] -> w705
                      tunnel: w704 -> [w796 w809]
                      tunnel: [w795 w804] -> w690
                      tunnel: [w794 w803] -> w689
                      tunnel: w688 -> [w794 w802]
                      tunnel: [w793 w801] -> w686
                      tunnel: w685 -> [w793 w800]
                      tunnel: [w795 w799] -> w684
                      tunnel: [w792 w798] -> w680
                      tunnel: w679 -> [w792 w797]
                      frame False {
                        w795 = 0
                      }
                      frame True {
                        n249 = Subtract(x=w811, y=w812) -> (x-y=w814:i32)
                        n250 = Array Subset(array=w810, index=w814, length=w812) -> (w815:dbl[])
                        "tvit (10 strides)" <- w815
                        n251 = call-poly <vilib>:"Mean.vi"("X"=w815) -> ("mean"=w813:dbl)  [unwired: 1 out]
                        "tvit (10 strides)" <- w813
                        n252 = Build Array (concatenate)(w809, w813) -> (w806:dbl[])
                        n253 = Array Size(array=w806) -> (size(s)=w805:i32)
                        n254 = Greater?(x=w805, y=10) -> (0:w807:bool)
                        n255 = case shown="True" w807 {
                          tunnel: w813 -> [_ w848]
                          tunnel: w806 -> [_ w841]
                          tunnel: w805 -> [_ _]
                          tunnel: [w819 w832] -> w804
                          tunnel: [w817 w828] -> w803
                          tunnel: w802 -> [w817 w824]
                          tunnel: [w818 w827] -> w801
                          tunnel: w800 -> [w818 w826]
                          tunnel: [w819 w825] -> w799
                          tunnel: [w816 w823] -> w798
                          tunnel: w797 -> [w816 w822]
                          frame False {
                            w819 = 0
                          }
                          frame True {
                            w830 = 10
                            w833 = 0
                            n256 = call "pr-ranking.vi"("element"=w848, "Database Array"=w841) -> ("PR Value"=w840:dbl)  [unwired: 1 out]
                            n257 = Array Size(array=w824) -> (size(s)=w844:i32)
                            n258 = Decrement(x=w844) -> (x-1=w843:i32)
                            n259 = Subtract(x=100, y=w840) -> (x-y=w821:dbl)
                            "TVItv SCORE" <- w821
                            n260 = Index Array(array=w824, index=w843) -> (element=w842:dbl)
                            n261 = Subtract(x=w821, y=w842) -> (x-y=→"10 STRIDE INCREMENT":dbl)
                            n262 = Build Array (concatenate)(w824, w821) -> (w828:dbl[])
                            n263 = Greater?(x=w821, y=95) -> (0:w834:bool)
                            n264 = Less?(x=w821, y=5) -> (x < y?=w835:bool)
                            n265 = Select(t=-2, s=w835, f=w833) -> (s? t:f=w837:i32)
                            n266 = Select(t=2, s=w834, f=w833) -> (s? t:f=w836:i32)
                            n267 = Add(x=w837, y=w836) -> (x+y=w832:i32)
                            n268 = Array Size(array=w828) -> (size(s)=w829:i32)
                            n269 = Greater?(x=w829, y=w830) -> (0:w831:bool)
                            n270 = case shown="True" w831 {
                              tunnel: w830 -> [_ w863]
                              tunnel: w829 -> [_ w862]
                              tunnel: w828 -> [_ w861]
                              tunnel: [w850 w857] -> w827
                              tunnel: w826 -> [w850 w855]
                              tunnel: [0 w856] -> w825
                              tunnel: [w849 w854] -> w823
                              tunnel: w822 -> [w849 w853]
                              frame False {
                              }
                              frame True {
                                n271 = Subtract(x=w862, y=w863) -> (x-y=w870:i32)
                                n272 = Array Subset(array=w861, index=w870, length=w863) -> (w867:dbl[])
                                n273 = for {
                                N: w863 -> [_]
                                tunnel: w870 -> [w889]
                                tunnel: [w888] -> w869 mode=indexing
                                i -> [w890]
                                n274 = Add(x=w889, y=w890) -> (x+y=w888:i32)
                                }
                                n275 = call <vilib>:"Linear Fit.vi"("Y"=w867, "X"=w869) -> ("Best Linear Fit"=w868:dbl[], "slope"=w852:dbl)  [unwired: 9 in, 3 out]
                                n276 = Bundle(w869, w867) -> (w865:cluster{i32[], dbl[]})  [unwired: 1 in]
                                n277 = Bundle(w869, "Best Linear Fit"=w868) -> (w866:cluster{i32[], "Best Linear Fit":dbl[]})  [unwired: 1 in]
                                n278 = Build Array (concatenate)(w855, w852) -> (w857:dbl[])
                                n279 = Array Size(array=w857) -> (size(s)=w860:i32)
                                n280 = Build Array(w866, w865) -> (→"10 Strides":cluster{i32[], "Best Linear Fit":dbl[]}[])
                                n281 = Greater?(x=w860, y=10) -> (0:w858:bool)
                                n282 = case shown="True" w858 {
                                tunnel: w857 -> [_ w876]
                                tunnel: w852 -> [_ w877]
                                tunnel: [0 w878] -> w856
                                tunnel: [w871 w874] -> w854
                                tunnel: w853 -> [w871 w875]
                                frame False {
                                }
                                frame True {
                                w885 = 0
                                n283 = call "pr-ranking.vi"("element"=w877, "Database Array"=w876) -> ("PR Value"=w874:dbl)  [unwired: 1 out]
                                "Slope SCORE" <- w874
                                n284 = Less?(x=w874, y=5) -> (x < y?=w880:bool)
                                n285 = Greater?(x=w874, y=95) -> (0:w879:bool)
                                n286 = Select(t=-2, s=w880, f=w885) -> (s? t:f=w882:i32)
                                n287 = Select(t=2, s=w879, f=w885) -> (s? t:f=w881:i32)
                                n288 = Add(x=w882, y=w881) -> (x+y=w878:i32)
                                n289 = Subtract(x=w874, y=w875) -> (x-y=→"10 SLOPE INCREMENT":dbl)
                                }
                                }
                              }
                            }
                          }
                        }
                      }
                    }
                    n290 = Add(x=w698, y=w697) -> (x+y=w694:i32)
                    n291 = Add(x=w690, y=w682) -> (x+y=w687:i32)
                    n292 = Add(x=w692, y=w691) -> (x+y=w693:i32)
                    n293 = Add(x=w684, y=w681) -> (x+y=w683:i32)
                  }
                }
                n294 = case shown="True" w573 {
                  tunnel: w572 -> [_ w622]
                  tunnel: w571 -> [_ w618]
                  tunnel: [w593 w601] -> w567
                  tunnel: w568 -> [w593 w606]
                  tunnel: [w591 w609] -> w566
                  tunnel: w559 -> [w592 w600]
                  tunnel: [w592 w599] -> w558
                  tunnel: [w591 w598] -> w557
                  tunnel: [w590 w597] -> w538
                  tunnel: w537 -> [w590 w596]
                  frame False {
                    w591 = 0
                  }
                  frame True {
                    w603 = 10
                    w614 = 0
                    n295 = call "pr-ranking.vi"("element"=w622, "Database Array"=w618) -> ("PR Value"=w621:dbl)  [unwired: 1 out]
                    n296 = Array Size(array=w606) -> (size(s)=w608:i32)
                    n297 = Subtract(x=100, y=w621) -> (x-y=w594:dbl)
                    "TVItv SCORE" <- w594
                    n298 = Decrement(x=w608) -> (x-1=w607:i32)
                    n299 = Index Array(array=w606, index=w607) -> (element=w605:dbl)
                    n300 = Subtract(x=w594, y=w605) -> (x-y=→"1 STRIDE INCREMENT":dbl)
                    n301 = Less?(x=w594, y=5) -> (x < y?=w616:bool)
                    n302 = Greater?(x=w594, y=95) -> (0:w615:bool)
                    n303 = Build Array (concatenate)(w606, w594) -> (w601:dbl[])
                    n304 = global write "tvi_arx_ni9234_global.vi" "1 stride boolean"(w615) -> ()
                    n305 = Select(t=-2, s=w616, f=w614) -> (s? t:f=w611:i32)
                    n306 = Select(t=2, s=w615, f=w614) -> (s? t:f=w610:i32)
                    n307 = Add(x=w611, y=w610) -> (x+y=w609:i32)
                    n308 = Array Size(array=w601) -> (size(s)=w604:i32)
                    n309 = Greater?(x=w604, y=w603) -> (0:w602:bool)
                    n310 = case shown="True" w602 {
                      tunnel: w603 -> [_ w637]
                      tunnel: w604 -> [_ w636]
                      tunnel: w601 -> [_ w635]
                      tunnel: [w625 w630] -> w599
                      tunnel: w600 -> [w625 w634]
                      tunnel: [0 w629] -> w598
                      tunnel: [w623 w627] -> w597
                      tunnel: w596 -> [w623 w626]
                      frame False {
                      }
                      frame True {
                        n311 = Subtract(x=w636, y=w637) -> (x-y=w638:i32)
                        n312 = Array Subset(array=w635, index=w638, length=w637) -> (w641:dbl[])
                        n313 = for {
                          N: w637 -> [_]
                          tunnel: w638 -> [w663]
                          tunnel: [w662] -> w640 mode=indexing
                          i -> [w664]
                          n314 = Add(x=w663, y=w664) -> (x+y=w662:i32)
                        }
                        n315 = call <vilib>:"Linear Fit.vi"("Y"=w641, "X"=w640) -> ("Best Linear Fit"=w639:dbl[], "slope"=w628:dbl)  [unwired: 9 in, 3 out]
                        n316 = Bundle(w640, w641) -> (w642:cluster{i32[], dbl[]})  [unwired: 1 in]
                        n317 = Bundle(w640, "Best Linear Fit"=w639) -> (w643:cluster{i32[], "Best Linear Fit":dbl[]})  [unwired: 1 in]
                        n318 = Build Array(w643, w642) -> (→"1 Stride":cluster{i32[], "Best Linear Fit":dbl[]}[])
                        n319 = Build Array (concatenate)(w634, w628) -> (w630:dbl[])
                        n320 = Array Size(array=w630) -> (size(s)=w633:i32)
                        n321 = Greater?(x=w633, y=10) -> (0:w631:bool)
                        n322 = case shown="True" w631 {
                          tunnel: w630 -> [_ w661]
                          tunnel: w628 -> [_ w650]
                          tunnel: [0 w651] -> w629
                          tunnel: [w645 w648] -> w627
                          tunnel: w626 -> [w645 w649]
                          frame False {
                          }
                          frame True {
                            w658 = 0
                            n323 = call "pr-ranking.vi"("element"=w650, "Database Array"=w661) -> ("PR Value"=w648:dbl)  [unwired: 1 out]
                            "Slope SCORE" <- w648
                            n324 = Less?(x=w648, y=5) -> (x < y?=w653:bool)
                            n325 = Greater?(x=w648, y=95) -> (0:w652:bool)
                            n326 = Select(t=-2, s=w653, f=w658) -> (s? t:f=w655:i32)
                            n327 = Select(t=2, s=w652, f=w658) -> (s? t:f=w654:i32)
                            n328 = Add(x=w655, y=w654) -> (x+y=w651:i32)
                            n329 = Subtract(x=w648, y=w649) -> (x-y=→"1 SLOPE INCREMENT":dbl)
                          }
                        }
                      }
                    }
                  }
                }
                n330 = Add(x=w566, y=w565) -> (x+y=w564:i32)
                n331 = Add(x=w557, y=w562) -> (x+y=w563:i32)
              }
            }
            n332 = for {
              tunnel: [w515] -> w459 mode=indexing
              tunnel: w450 -> [_] mode=indexing
              i -> [w516]
              n333 = To Double Precision Float(number=w516) -> (double precision float=w515:dbl)
            }
            n334 = Array Subset(array=w461, index=w444, length=w452) -> (w466:dbl[])
            n335 = Array Subset(array=w460, index=w444, length=w452) -> (w465:dbl[])
            n336 = global write "tvi_arx_ni9234_global.vi" "step-interval"(w452) -> ()
            n337 = Divide(x=w452, y=w458) -> (x/y=→"CURRENT STEP INTERVAL (sec)":dbl)
            n338 = Divide(x=w459, y=w458) -> (x/y=w451:dbl[])
            n339 = Add Array Elements(numeric array=w466) -> (sum=w463:dbl)
            n340 = Add Array Elements(numeric array=w465) -> (sum=w464:dbl)
            n341 = Greater?(x=w463, y=w464) -> (0:w462:bool)
            n342 = Bundle(w451, w450) -> (w448:cluster{dbl[], dbl[]})  [unwired: 1 in]
            n343 = Build Array(w447, w448) -> (w453:cluster{dbl[], dbl[]}[])
            n344 = Less?(x=w455, y=w454) -> (x < y?=w457:bool)
            n345 = case shown="False" w462 {
              tunnel: w453 -> [w517 w518]
              frame False {
                "Right Foot GRF" <- w517
              }
              frame True {
                "Left Foot GRF" <- w518
              }
            }
            n346 = case shown="False" w457 {
              tunnel: [w512 w514] -> w456
              tunnel: w455 -> [_ w514]
              tunnel: w454 -> [w512 _]
              tunnel: [w511 w513] -> w449
              tunnel: w447 -> [w511 _]
              tunnel: w448 -> [_ w513]
              frame False {
              }
              frame True {
              }
            }
          }
        }
        n347 = for {
          tunnel: [w417] -> w383 mode=indexing
          tunnel: w376 -> [_] mode=indexing
          i -> [w418]
          n348 = To Double Precision Float(number=w418) -> (double precision float=w417:dbl)
        }
        n349 = for {
          tunnel: [w420] -> w388 mode=indexing
          tunnel: w382 -> [w420] mode=indexing
          tunnel: [1.0] -> w387 mode=indexing
        }
        n350 = Bundle(w383, w376) -> (w385:cluster{dbl[], dbl[]})  [unwired: 1 in]
        n351 = Bundle(w388, w387) -> (w386:cluster{dbl[], dbl[]})  [unwired: 1 in]
        n352 = Build Array(w385, w386) -> (→"GRF Input":cluster{dbl[], dbl[]}[])
      }
      frame True {
        w903 = 2  # 2(sec)
        n353 = Multiply(x=w904, y=w903) -> (x*y=w940:i32)
        n354 = Divide(x=w904, y=w903) -> (x/y=w905:dbl)
        n355 = Subtract(x=w924, y=w940) -> (x-y=w926:dbl)
        n356 = Array Subset(array=w932, index=w926, length=w940) -> (w941:dbl[])
        n357 = call <vilib>:"Std Deviation and Variance.vi"("X"=w941) -> ("standard deviation"=w944:dbl)  [unwired: 1 in, 2 out]
        "std(loadcell)" <- w944
        n358 = Greater?(x=w944, y=0.7 ("標準差門檻值")) -> (0:w933:bool)
        n359 = case shown="True" w933 {
          tunnel: w947 -> [w993 w998]
          tunnel: [w994 w997] -> w930
          tunnel: w905 -> [_ w995]
          frame False {
            n360 = Multiply(x=0, y=w993) -> (x*y=w994:dbl)
          }
          frame True {
            n361 = Increment(x=w998) -> (x+1=w997:dbl)
            n362 = global write "tvi_arx_ni9234_global.vi" "standstill boolean"(FALSE) -> ()
            n363 = global write "tvi_arx_ni9234_global.vi" "step-interval"(w995) -> ()
          }
        }
        n364 = Equal?(x=w930, y=64) -> (x = y?=w945:bool)
        n365 = Equal?(x=w930, y=144) -> (x = y?=w929:bool)
        n366 = case shown="True" w929 {
          tunnel: [0 w954] -> w928
          tunnel: w904 -> [_ w962]
          tunnel: w927 -> [_ w953]
          tunnel: w924 -> [_ w963]
          frame False {
          }
          frame True {
            w964 = 8  # 8(sec)
            n367 = Multiply(x=w964, y=w962) -> (x*y=w966:i32)
            n368 = Subtract(x=w963, y=w966) -> (x-y=w965:dbl)
            n369 = Array Subset(array=w953, index=w965, length=w966) -> (w950:dbl[])
            n370 = call "z-score.vi"("Array"=w950) -> ("Z-Score"=w952:dbl[])  [unwired: 2 out]
            n371 = call "indexing_steps.vi"("z-score series (input)"=w952) -> ("index of step (output)"=w951:dbl[])  [unwired: 5 in]
            n372 = Array Size(array=w951) -> (size(s)=w957:i32)
            n373 = Decrement(x=w957) -> (x-1=w955:i32)
            n374 = Index Array(array=w951, index=w955) -> (element=w961:dbl)
            n375 = Index Array(array=w951, index=0) -> (element=w960:dbl)
            n376 = Subtract(x=w961, y=w960) -> (x-y=w959:dbl)
            n377 = Array Subset(array=w950, index=w960, length=w959) -> (w958:dbl[])
            n378 = call-poly <vilib>:"Mean.vi"("X"=w958) -> ("mean"=w954:dbl)  [unwired: 1 out]
          }
        }
        n379 = case shown="True" w945 {
          tunnel: w932 -> [_ w977]
          tunnel: w924 -> [_ w975]
          tunnel: w904 -> [_ w973]
          tunnel: [0 w969] -> w925
          frame False {
          }
          frame True {
            w976 = 8  # 8(sec)
            n380 = Multiply(x=w976, y=w973) -> (x*y=w972:i32)
            n381 = Subtract(x=w975, y=w972) -> (x-y=w974:dbl)
            n382 = Array Subset(array=w977, index=w974, length=w972) -> (w968:dbl[])
            n383 = Sort 1D Array(array=w968) -> (sorted array=w971:dbl[])
            n384 = while {
              tunnel: w971 -> [w978]
              tunnel: 8 -> [w980]
              tunnel: [w984] -> w969
              i -> [w983]
              stop <- w990 stop-if-true
              n385 = Increment(x=w983) -> (x+1=w981:i32)
              n386 = Multiply(x=w981, y=w980) -> (x*y=w979:i32)
              n387 = Multiply(x=w980, y=w983) -> (x*y=w982:i32)
              n388 = Array Subset(array=w978, index=w979, length=w980) -> (w989:dbl[])
              n389 = Array Subset(array=w978, index=w982, length=w980) -> (w988:dbl[])
              n390 = call-poly <vilib>:"Mean.vi"("X"=w988) -> ("mean"=w986:dbl)  [unwired: 1 out]
              n391 = call-poly <vilib>:"Mean.vi"("X"=w989) -> ("mean"=w987:dbl)  [unwired: 1 out]
              n392 = Subtract(x=w987, y=w986) -> (x-y=w985:dbl)
              n393 = Greater?(x=w985, y=-5e-05) -> (0:w990:bool)
              n394 = Index Array(array=w978, index=w979) -> (element=w984:dbl)
            }
          }
        }
        n395 = Add(x=w928, y=w943) -> (x+y=w942:dbl)
      }
    }
    "window start index" <- w305
    n396 = Add(x=w287, y=w289) -> (x+y=w288:dbl)
    "new step interval in last loop" <- w291
    "new step index(global) in last loop" <- w292
    "main loop" <- w157
    "mean" <- w300
    "baseline value" <- w287
  }
  n397 = Concatenate Strings("Name", ".txt" ("time format string (%c)")) -> (w11:string)
  n398 = Build Path(base path=path "F:/DAQ/GRF" ("Path 2"), name or relative path=w11) -> (appended path=w23:path)
  n399 = Build Path(base path=path "F:/DAQ/ECG" ("Path 2"), name or relative path=w11) -> (appended path=w10:path)
  n400 = while {
    tunnel: w5 -> [w1009]
    tunnel: w6 -> [w1008]
    tunnel: [w1007] -> w19
    tunnel: [w1006] -> w18
    shift-right: [w1001] -> _
    shift-left: 0 -> [w1005]
    shift-right: [w1004] -> _
    shift-left: TRUE -> [w1000]
    tunnel: w23 -> [w1002]
    tunnel: w10 -> [w999]
    i -> [w1003]
    stop <- w1000 continue-if-true
    n401 = case shown="True" w1000 {
      tunnel: w1009 -> [w1012 w1025]
      tunnel: w1008 -> [w1011 w1024]
      tunnel: [w1012 w1023] -> w1007
      tunnel: [w1011 w1022] -> w1006
      tunnel: w1005 -> [w1010 w1019]
      tunnel: [_ w1018] -> w1004
      tunnel: w1003 -> [_ w1017]
      tunnel: w1002 -> [_ w1015]
      tunnel: [w1010 w1014] -> w1001
      tunnel: w999 -> [_ w1013]
      frame False {
      }
      frame True {
        n402 = Dequeue Element(queue=w1025, error in (no error)=w1024) -> (queue out=w1023:refnum<queue>, element=w1021:cluster{"DataArray":dbl[][], "Recording":bool}, error out=w1022:errorcluster)  [unwired: 1 in, 1 out]
        n403 = Unbundle By Name(w1021) -> ("DataArray"=w1020:dbl[][], "Recording"=w1018:bool)
        n404 = Not Equal To 0?(x=w1017) -> (x != 0?=w1016:bool)
        n405 = case shown="True" w1016 {
          tunnel: w1020 -> [_ w1031]
          tunnel: w1015 -> [_ w1030]
          tunnel: [w1026 w1045] -> w1014
          tunnel: w1019 -> [w1026 w1044]
          tunnel: w1013 -> [_ w1027]
          frame False {
          }
          frame True {
            n406 = Array Subset(array=w1031, index (col)=0, length (col)=4) -> (w1034:dbl[][])  [unwired: 2 in]
            n407 = Array Subset(array=w1031, index (col)=4, length (col)=1) -> (w1029:dbl[][])  [unwired: 2 in]
            n408 = Array Size(array=w1031) -> (size(s)=w1041:i32[])
            n409 = call-poly <vilib>:"Write To Spreadsheet File.vi"("format (%.3f)"="%7f", "append to file? (new file:F)"=TRUE, "2D data"=w1034, "file path (dialog if empty)"=w1030) -> ("new file path (Not A Path if cancelled)"=→"GRF File":path)  [unwired: 4 in]
            n410 = call-poly <vilib>:"Write To Spreadsheet File.vi"("format (%.3f)"="%7f", "append to file? (new file:F)"=TRUE, "2D data"=w1029, "file path (dialog if empty)"=w1027) -> ("new file path (Not A Path if cancelled)"=→"ECG File":path)  [unwired: 4 in]
            n411 = Index Array(array=w1041) -> (element=w1040:i32)  [unwired: 1 in]
            n412 = Add(x=w1040, y=w1044) -> (x+y=w1045:i32)
          }
        }
        "file length" <- w1014
      }
    }
    "Recording" <- w1000
  }
  n413 = Release Queue(queue=w19, force destroy? (F)=TRUE, error in (no error)=w18) -> (error out=w21:errorcluster)  [unwired: 2 out]
  n414 = call <vilib>:"Simple Error Handler.vi"("error in (no error)"=w21) -> ()  [unwired: 4 in, 5 out]
  "running phase" <- w41
